vi "YKMW100 Module Filter.vi"(8 "Error In":errorcluster, 10 "Select Module":string="1 ", 11 "All Data Input":string[](array[string])) -> (0 "Error Out":errorcluster, 2 "Specific Point":string, 3 "All Data Output":string[](array[string]))   [LabVIEW 2016]
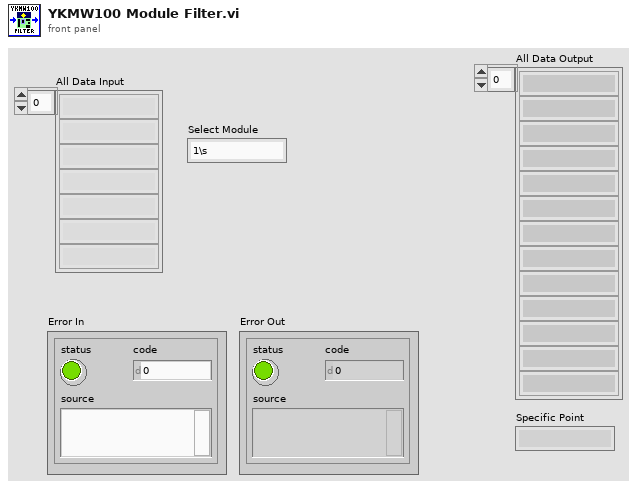
[diagram p1: front panel]
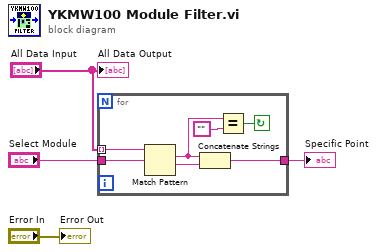
[diagram p0: block diagram]
diagram:
  n1 = for {
    tunnel: "All Data Input" -> [w11] mode=indexing
    tunnel: [w9] -> w4
    tunnel: "Select Module" -> [w5]
    stop <- w8 continue-if-true
    n2 = Match Pattern(string=w11, regular expression=w5) -> (match substring=w7:string, after substring=w10:string)  [unwired: 1 in, 2 out]
    n3 = Concatenate Strings(w7, w10) -> (w9:string)
    n4 = Equal?(x=w7, y="") -> (x = y?=w8:bool)
  }
  "Specific Point" <- w4
  "Error Out" <- "Error In"
  "All Data Output" <- "All Data Input"
